vi "Get TypeDef Info From Bitfile.vi"(8 "error in":errorcluster, 11 "Bitfile Path":path) -> (0 "error out":errorcluster, 3 "TypeDef Info":cluster{string, cluster{"Name":string, i32}[]}[](array[cluster]))   [LabVIEW 2010]
uses:
  <userlib>/_FPGA Interface Advanced Tools/FPGA Bitfile Utility/TypeDefs/Control_Indicator Info.ctl
  <vilib>/rvi/DataTransferAndStorage/Container/Common/niFpgaDataTypeControl.ctl
  <userlib>/_FPGA Interface Advanced Tools/FPGA Bitfile Utility/TypeDefs/FIFO Info.ctl
  <userlib>/_FPGA Interface Advanced Tools/FPGA Bitfile Utility/FPGA Bitfile Utility.lvlib
panel:
  out "HostToTarget":cluster{T1[]}[](array[cluster])
  out "TargetToHost":cluster{T1[]}[](array[cluster])
  out "Control Scalars":cluster{T3[]}[](array[cluster])
  out "Control Arrays":cluster{T3[]}[](array[cluster])
  out "Indicator Arrays":cluster{T3[]}[](array[cluster])
  out "Indicator Scalars":cluster{T3[]}[](array[cluster])
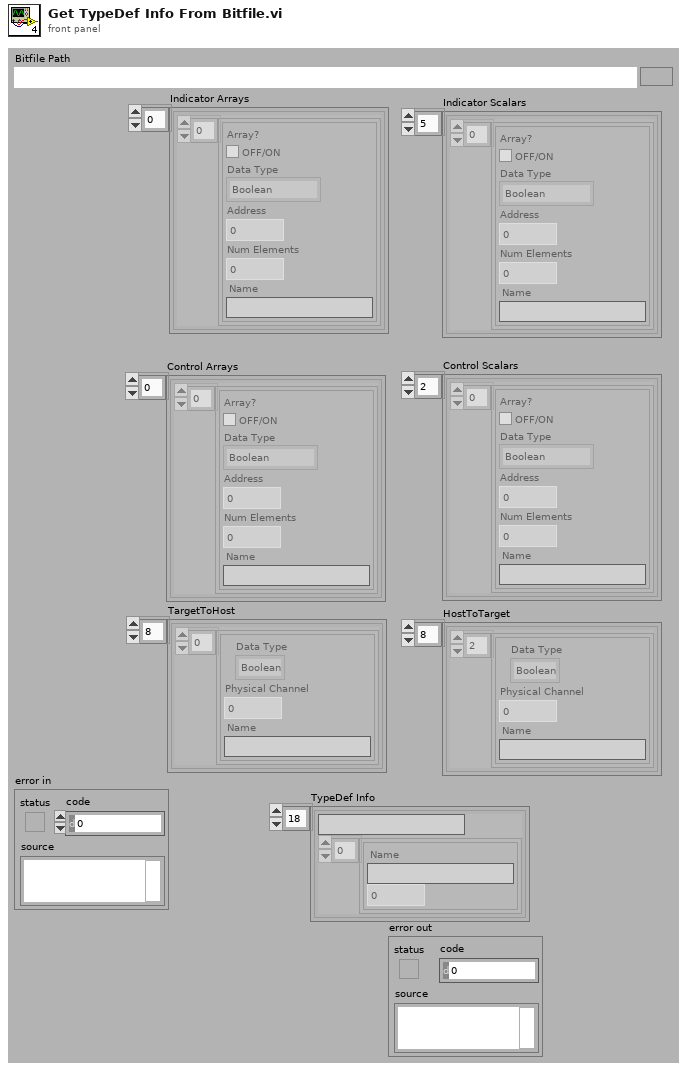
[diagram p1: front panel]
types:
  T1 = typedef "FPGA Bitfile Utility.lvlib/FIFO Info.ctl" = cluster{"Data Type":T2, "Physical Channel":u32, "Name":string}
  T2 = typedef "niFpgaDataTypeControl.ctl" = enum32{"Boolean", "I8", "I16", "I32", "I64", "U8", "U16", "U32", "U64", "FXP", "CustomControl"}
  T3 = typedef "FPGA Bitfile Utility.lvlib/Control_Indicator Info.ctl" = cluster{"Array?":bool, "Data Type":T2, "Address":u32, "Num Elements":u32, "Name":string}
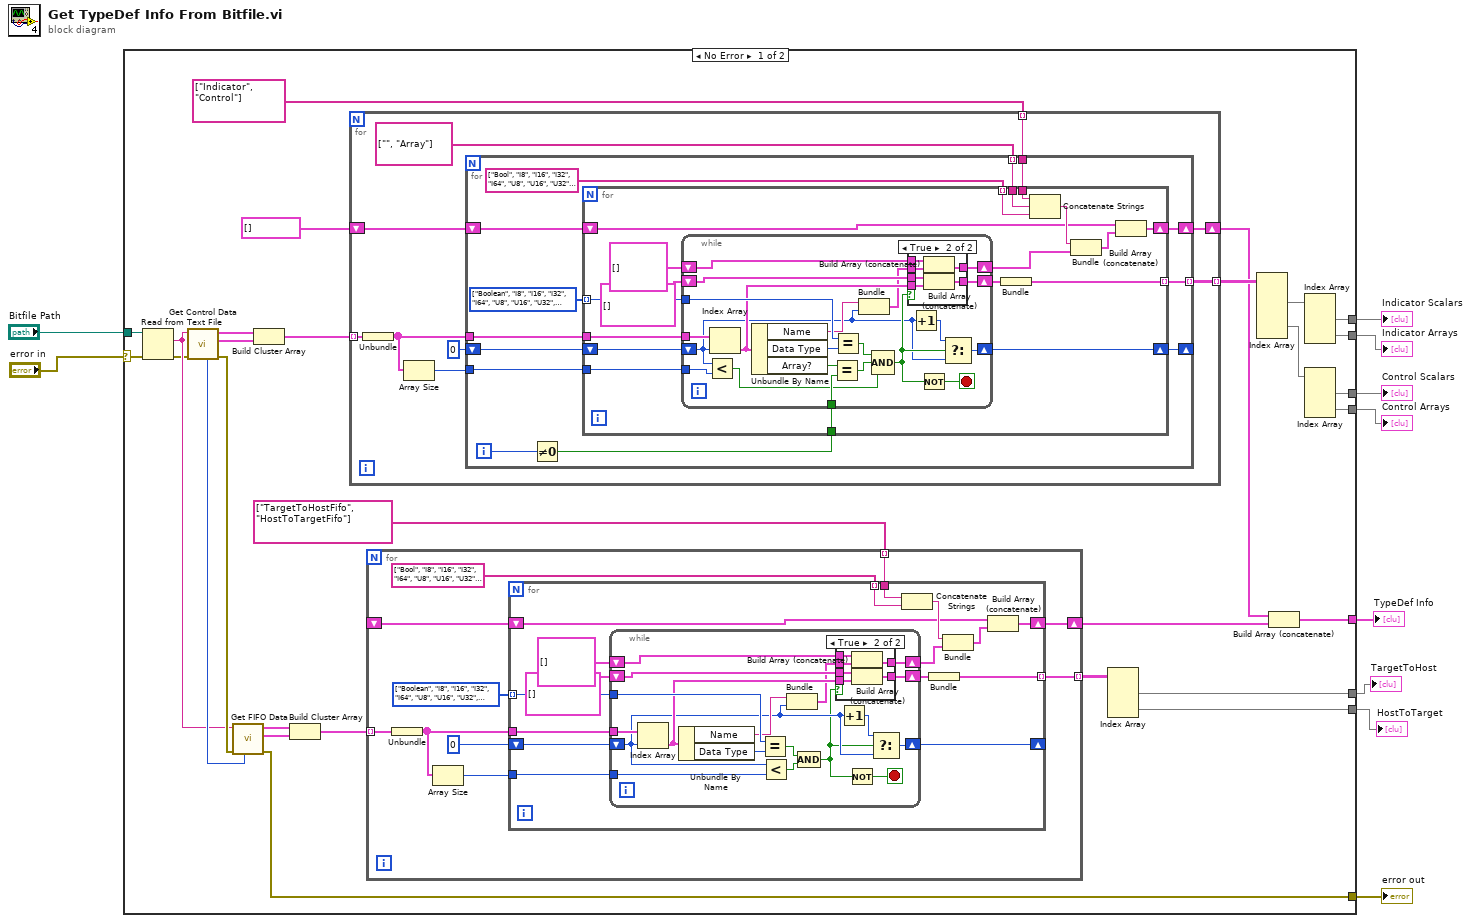
[diagram p0: block diagram]
diagram:
  n1 = case shown="No Error" "error in" {
    selector: "error in" -> [w11 w161]
    tunnel: "Bitfile Path" -> [w37 _]
    tunnel: [w19 _] -> w9
    tunnel: [w18 _] -> w8
    tunnel: [w17 _] -> w7
    tunnel: [w16 _] -> w6
    tunnel: [w15 _] -> w5
    tunnel: [w14 _] -> w4
    tunnel: [w13 _] -> w3
    tunnel: [w12 w161] -> w2
    frame No Error {
      n2 = Read from Text File(file (use dialog)=w37, error in=w11) -> (text=w36:string, error out=w35:errorcluster)  [unwired: 4 out]
      n3 = call <userlib>:"Get Control Data.vi"("error in (no error)"=w35, "bitfile xml in"=w36) -> ("error out"=w38:errorcluster, "Controls"=w22:T3[], "Indicators"=w23:T3[], "offset past EndTag"=w39:i32)  [unwired: 6 in]
      n4 = call <userlib>:"Get FIFO Data.vi"("offset"=w39, "error in (no error)"=w38, "bitfile xml in"=w36) -> ("error out"=w12:errorcluster, "HostToTargetFIFOs"=w20:T1[], "TargetToHost FIFOs"=w21:T1[])  [unwired: 5 in, 1 out]
      n5 = Build Cluster Array(w23, w22) -> (w34:cluster{"Controls":T3[]}[])
      n6 = Build Cluster Array(w21, w20) -> (w28:cluster{"HostToTargetFIFOs":T1[]}[])
      n7 = for {
        tunnel: w34 -> [w100] mode=indexing
        tunnel: [w99] -> w33 mode=indexing
        tunnel: string[] ["Indicator", "Control"] -> [w97] mode=indexing
        shift-right: [w96] -> w25
        shift-left: cluster{string, cluster{"Name":string, i32}[]}[] [] -> [w95]
        n8 = Unbundle(w100) -> ("Controls"=w93:T3[])
        n9 = Array Size(array=w93) -> (size(s)=w92:i32)
        n10 = for {
          tunnel: w93 -> [w113]
          shift-right: [w110] -> _
          shift-left: 0 -> [w111]
          tunnel: [w108] -> w99 mode=indexing
          tunnel: string[] ["", "Array"] -> [w104] mode=indexing
          tunnel: w97 -> [w105]
          shift-right: [w103] -> w96
          shift-left: w95 -> [w102]
          tunnel: w92 -> [w101]
          i -> [w112]
          w107 = T2[] [enum."Boolean", enum."I8", enum."I16", enum."I32", enum."I64", enum."U8", enum."U16", enum."U32", enum."U64"] items=["Boolean", "I8", "I16", "I32", "I64", "U8", "U16", "U32", "U64", "FXP", "CustomControl"]
          n11 = Not Equal To 0?(x=w112) -> (x != 0?=w109:bool)
          n12 = for {
            tunnel: w107 -> [w131] mode=indexing
            tunnel: w113 -> [w130]
            tunnel: w109 -> [w127]
            shift-right: [w128] -> w110
            shift-left: w111 -> [w129]
            tunnel: [w124] -> w108 mode=indexing
            tunnel: string[] ["Bool", "I8", "I16", "I32", "I64", "U8", "U16", "U32", "U64"] -> [w119] mode=indexing
            tunnel: w105 -> [w121]
            tunnel: w104 -> [w120]
            shift-right: [w116] -> w103
            shift-left: w102 -> [w115]
            tunnel: w101 -> [w114]
            n13 = while {
              tunnel: w131 -> [w146]
              tunnel: w130 -> [w152]
              shift-right: [w150] -> w128
              shift-left: w129 -> [w134]
              tunnel: w127 -> [w148]
              shift-right: [w142] -> w126
              shift-left: T3[] [] -> [w141]
              shift-right: [w135] -> w122
              shift-left: cluster{"Name":string, i32}[] [] -> [w137]
              tunnel: w114 -> [w133]
              stop <- w139 stop-if-true
              n14 = Less?(x=w134, y=w133) -> (x < y?=w132:bool)
              n15 = Index Array(array=w152, index=w134) -> (element=w143:T3)
              n16 = Unbundle By Name(w143) -> ("Name"=w138:string, "Data Type"=w147:T2, "Array?"=w149:bool)
              n17 = Equal?(x=w149, y=w148) -> (x = y?=w145:bool)
              n18 = Equal?(x=w146, y=w147) -> (x = y?=w144:bool)
              n19 = Bundle("Name"=w138, w134) -> (w136:cluster{"Name":string, i32})  [unwired: 1 in]
              n20 = Compound Arithmetic op=AND(w144, w145, w132) -> (w140:bool)
              n21 = case shown="True" w140 {
                tunnel: w143 -> [_ w160]
                tunnel: [w154 w159] -> w142
                tunnel: w141 -> [w154 w158]
                tunnel: w137 -> [w153 w157]
                tunnel: w136 -> [_ w156]
                tunnel: [w153 w155] -> w135
                frame False {
                }
                frame True {
                  n22 = Build Array (concatenate)(w157, w156) -> (w155:cluster{"Name":string, i32}[])
                  n23 = Build Array (concatenate)(w158, w160) -> (w159:T3[])
                }
              }
              n24 = Increment(x=w134) -> (x+1=w151:i32)
              n25 = Not(x=w140) -> (.not. x?=w139:bool)
              n26 = Select(t=w151, s=w140, f=w134) -> (s? t:f=w150:i32)
            }
            n27 = Bundle(w126) -> (w124:cluster{T3[]})  [unwired: 1 in]
            n28 = Concatenate Strings(w121, w120, w119) -> (w118:string)
            n29 = Bundle(w118, w122) -> (w117:cluster{string, cluster{"Name":string, i32}[]})  [unwired: 1 in]
            n30 = Build Array (concatenate)(w115, w117) -> (w116:cluster{string, cluster{"Name":string, i32}[]}[])
          }
        }
      }
      n31 = for {
        tunnel: w28 -> [w49] mode=indexing
        tunnel: [w48] -> w26 mode=indexing
        shift-right: [w47] -> w24
        shift-left: _ -> [w46]
        tunnel: string[] ["TargetToHostFifo", "HostToTargetFifo"] -> [w43] mode=indexing
        w45 = T2[] [enum."Boolean", enum."I8", enum."I16", enum."I32", enum."I64", enum."U8", enum."U16", enum."U32", enum."U64"] items=["Boolean", "I8", "I16", "I32", "I64", "U8", "U16", "U32", "U64", "FXP", "CustomControl"]
        n32 = Unbundle(w49) -> ("HostToTargetFIFOs"=w40:T1[])
        n33 = Array Size(array=w40) -> (size(s)=w41:i32)
        n34 = for {
          tunnel: w45 -> [w65] mode=indexing
          tunnel: w40 -> [w64]
          shift-right: [w62] -> _
          shift-left: 0 -> [w63]
          tunnel: [w60] -> w48 mode=indexing
          tunnel: string[] ["Bool", "I8", "I16", "I32", "I64", "U8", "U16", "U32", "U64"] -> [w56] mode=indexing
          tunnel: w43 -> [w57]
          shift-right: [w53] -> w47
          shift-left: w46 -> [w52]
          tunnel: w41 -> [w50]
          n35 = while {
            tunnel: w65 -> [w79]
            tunnel: w64 -> [w83]
            shift-right: [w81] -> w62
            shift-left: w63 -> [w69]
            shift-right: [w77] -> w61
            shift-left: T1[] [] -> [w76]
            shift-right: [w71] -> w58
            shift-left: cluster{"Name":string, i32}[] [] -> [w73]
            tunnel: w50 -> [w70]
            stop <- w75 stop-if-true
            n36 = Index Array(array=w83, index=w69) -> (element=w78:T1)
            n37 = Unbundle By Name(w78) -> ("Name"=w74:string, "Data Type"=w80:T2)
            n38 = Equal?(x=w79, y=w80) -> (x = y?=w67:bool)
            n39 = Less?(x=w69, y=w70) -> (x < y?=w68:bool)
            n40 = Bundle("Name"=w74, w69) -> (w72:cluster{"Name":string, i32})  [unwired: 1 in]
            n41 = Compound Arithmetic op=AND(w67, w68) -> (w66:bool)
            n42 = case shown="True" w66 {
              tunnel: w78 -> [_ w91]
              tunnel: [w85 w90] -> w77
              tunnel: w76 -> [w85 w89]
              tunnel: w73 -> [w84 w88]
              tunnel: w72 -> [_ w87]
              tunnel: [w84 w86] -> w71
              frame False {
              }
              frame True {
                n43 = Build Array (concatenate)(w88, w87) -> (w86:cluster{"Name":string, i32}[])
                n44 = Build Array (concatenate)(w89, w91) -> (w90:T1[])
              }
            }
            n45 = Increment(x=w69) -> (x+1=w82:i32)
            n46 = Not(x=w66) -> (.not. x?=w75:bool)
            n47 = Select(t=w82, s=w66, f=w69) -> (s? t:f=w81:i32)
          }
          n48 = Concatenate Strings(w57, w56) -> (w55:string)
          n49 = Bundle(w61) -> (w60:cluster{T1[]})  [unwired: 1 in]
          n50 = Bundle(w55, w58) -> (w54:cluster{string, cluster{"Name":string, i32}[]})  [unwired: 1 in]
          n51 = Build Array (concatenate)(w52, w54) -> (w53:cluster{string, cluster{"Name":string, i32}[]}[])
        }
      }
      n52 = Index Array(array=w26) -> (element #1=w18:cluster{T1[]}[], element #2=w17:cluster{T1[]}[])  [unwired: 4 in]
      n53 = Index Array(array=w33) -> (element #1=w32:cluster{T3[]}[][], element #2=w31:cluster{T3[]}[][])  [unwired: 6 in]
      n54 = Build Array (concatenate)(w25, w24) -> (w19:cluster{string, cluster{"Name":string, i32}[]}[])
      n55 = Index Array(array=w32) -> (element #1=w13:cluster{T3[]}[], element #2=w14:cluster{T3[]}[])  [unwired: 4 in]
      n56 = Index Array(array=w31) -> (element #1=w15:cluster{T3[]}[], element #2=w16:cluster{T3[]}[])  [unwired: 4 in]
    }
    frame Error {
    }
  }
  "Indicator Scalars" <- w3
  "Indicator Arrays" <- w4
  "Control Scalars" <- w5
  "Control Arrays" <- w6
  "TypeDef Info" <- w9
  "TargetToHost" <- w8
  "HostToTarget" <- w7
  "error out" <- w2
